vi "collectCI2_img.vi"() -> (0 "Avg cts/s":dbl, 1 "recorded samples":i32, 2 "wrap":i32)   [LabVIEW 2013]
uses:
  <vilib>/DAQmx/read.llb/DAQmx Read (Counter 1D U32 1Chan NSamp).vi
  <vilib>/DAQmx/miscellaneous.llb/DAQmx Fill In Error Info.vi
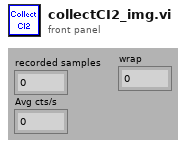
[diagram p1: front panel]
types:
  T1 = typedef "LVRectTypeDef.ctl" = cluster{"Left":i16, "Top":i16, "Right":i16, "Bottom":i16}
  T2 = cluster{"Xpixels":i32, "Vxminref":dbl, "Vxmaxref":dbl, "P":dbl, "Ypixels":i32, "Vyminref":dbl, "Vymaxref":dbl, "srate":sgl, "sAOxy":i32, "timeout":dbl, "type":string, "date":string, "time":string, "Colormap":u16, "Drawing Mode":u16, "Scanning Mode":u16, "square pixels":bool, "square matrix":bool, "Xpixels Img":i32, "Vx-min Img":dbl, "VX-max Img":dbl, "Ypixels Img":i32, "Vy-min Img":dbl, "Vy-max Img ":dbl, "Angle Img":dbl, "autoshutter":bool, "finite":bool, "cont":bool, "wavdet":bool, "measpoints":i32, "avpp":i32, "bufferAO":i32, "bufferAI":i32, "CH1":bool, "CH2":bool, "X":bool, "Y":bool, "Ip":bool, "Vp":bool, "starttick":u32, "waveform":path, "Vx-ref":dbl, "Vy-ref":dbl, "refreshrate":dbl, "refreshbuffer":i32, "tt_cycles":i32, "motorref":refnum<k7>, "mirrorswitch":refnum<k7>, "sample mode":i32, "maxbufferAI":i32, "sampletreshold":dbl, "srateAODO":sgl, "bin":sgl, "Pel":sgl, "Angle draw":dbl, "srate Img":sgl, "ROIimg_plotbounds":T1, "auto OD":bool, "ODfilt":u16, "reset AO_DO":bool}
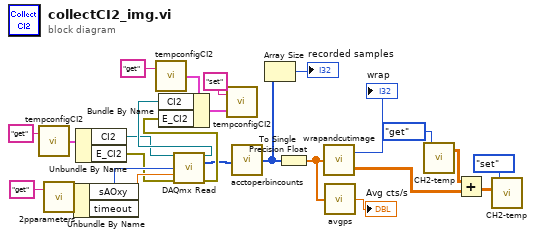
[diagram p0: block diagram]
diagram:
  n1 = call "tempconfigCI2.vi"("command"="get") -> ("Temp Config out"=w14:cluster{"CI2":refnum<k21>, "E_CI2":errorcluster})  [unwired: 1 in]
  n2 = call "2pparameters.vi"("command"="get") -> ("Params out"=w12:T2)  [unwired: 1 in]
  n3 = Unbundle By Name(w12) -> ("sAOxy"=w18:i32, "timeout"=w19:dbl)
  n4 = Unbundle By Name(w14) -> ("CI2"=w16:refnum<k21>, "E_CI2"=w17:errorcluster)
  n5 = call "tempconfigCI2.vi"("command"="get") -> ("Temp Config out"=w20:cluster{"CI2":refnum<k21>, "E_CI2":errorcluster})  [unwired: 1 in]
  n6 = call-poly <vilib>:"DAQmx Read.vi"("task/channels in"=w16, "number of samples per channel"=w18, "timeout"=w19, "error in"=w17) -> ("task out"=w25:refnum<k21>, "data"=w4:u32[], "error out"=w24:errorcluster)  [unwired: 9 in]
  n7 = Bundle By Name(cluster=w20, "CI2"=w25, "E_CI2"=w24) -> (w23:cluster{"CI2":refnum<k21>, "E_CI2":errorcluster})
  n8 = call "tempconfigCI2.vi"("Temp Config in"=w23, "command"="set") -> ()  [unwired: 1 out]
  n9 = call "acctoperbincounts.vi"("accumulative counts"=w4) -> ("counts per bin"=w5:u32[])
  n10 = Array Size(array=w5) -> (size(s)=→"recorded samples":i32)
  n11 = To Single Precision Float(number=w5) -> (single precision float=w6:sgl[])
  n12 = call "wrapandcutimage.vi"("rasterscanned array"=w6) -> ("imagearray"=w10:sgl[][], "wrap"=→"wrap":i32)
  n13 = call "avgps.vi"("data"=w6) -> ("Avg cts/s"=→"Avg cts/s":dbl)
  n14 = call "CH2-temp.vi"("command"=enum16{"get", "set", "clear", "add row"}."get") -> ("array out"=w9:sgl[][])  [unwired: 3 in, 1 out]
  n15 = Add(x=w9, y=w10) -> (x+y=w11:sgl[][])
  n16 = call "CH2-temp.vi"("array in"=w11, "command"=enum16{"get", "set", "clear", "add row"}."set") -> ()  [unwired: 2 in, 2 out]
